vi "Set Create Test Node List.vi"(8 "error in (no error)":errorcluster, 10 "Create Test Node List":string[](array[string]), 11 "Abstract Create Test Node List Msg in":refnum<class "Abstract Create Test Node List Msg.lvclass">) -> (0 "error out":errorcluster, 3 "Abstract Create Test Node List Msg out":refnum<class "Abstract Create Test Node List Msg.lvclass">)   [LabVIEW 2013, in "Create Test Node Model.lvlib" / "Abstract Create Test Node List Msg.lvclass"]
uses:
  Abstract Create Test Node List Msg.lvclass
  Abstract Create Test Node List Msg.lvclass/Abstract Create Test Node List Msg.ctl
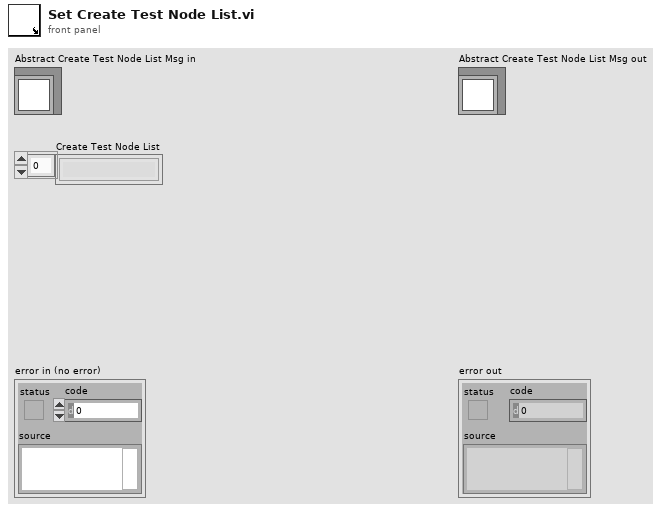
[diagram p1: front panel]
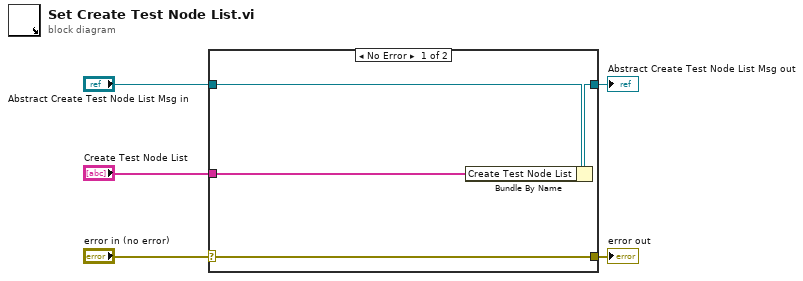
[diagram p0: block diagram]
diagram:
  n1 = case shown="No Error" "error in (no error)" {
    selector: "error in (no error)" -> [w9 w10]
    tunnel: [w9 w10] -> w4
    tunnel: [w7 w11] -> w2
    tunnel: "Abstract Create Test Node List Msg in" -> [w8 w11]
    tunnel: "Create Test Node List" -> [w6 _]
    frame No Error {
      n2 = Bundle By Name(cluster=w8, "Create Test Node List"=w6) -> (w7:refnum<class "Abstract Create Test Node List Msg.lvclass">)
    }
    frame Error {
    }
  }
  "error out" <- w4
  "Abstract Create Test Node List Msg out" <- w2
